vi "Read Data.vi"(7 "SPI Peripheral":refnum<class "SPI Peripheral.lvclass">, 8 "error in (no error)":errorcluster, 9 "Len":u8, 11 "Session In":refnum<class "Session.lvclass">) -> (0 "error out":errorcluster, 1 "Data":string, 3 "Session Out":refnum<class "Session.lvclass">)   [LabVIEW 2020, in "CTI.lvlib" / "SPI Peripheral.lvclass"]
uses:
  SPI Peripheral.lvclass
  Session/Session.lvclass
  SPI Peripheral.lvclass/SPI Peripheral.ctl
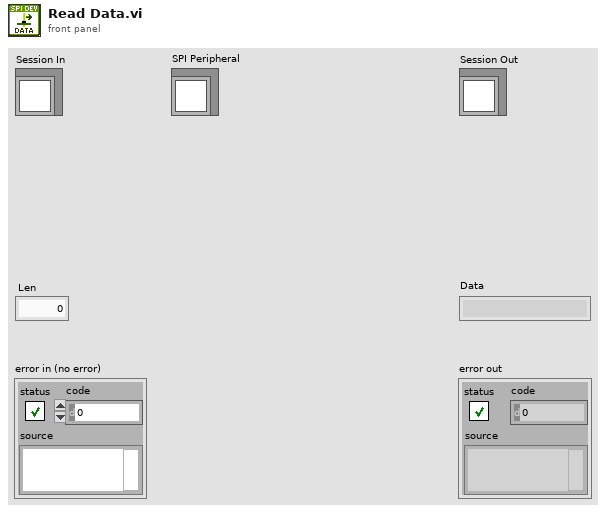
[diagram p1: front panel]
types:
  T1 = typedef "CTI.lvlib/SPI Number.ctl" = i8
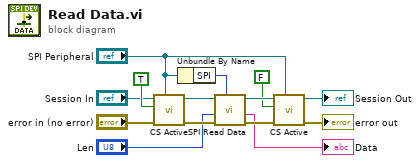
[diagram p0: block diagram]
diagram:
  n1 = call "CS Active.vi"("SPI Peripheral in"="SPI Peripheral", "error in (no error)"="error in (no error)", "CS Active"=TRUE, "Session In"="Session In") -> ("error out"=w12:errorcluster, "Session Out"=w8:refnum<class "Session.lvclass">)  [unwired: 6 in]
  n2 = Unbundle By Name("SPI Peripheral") -> ("SPI"=w11:T1)
  n3 = call "SPI Read Data.vi"("SPI #"=w11, "error in (no error)"=w12, "Len"="Len", "Session in"=w8) -> ("error out"=w13:errorcluster, "Data"=→"Data":string, "Session out"=w14:refnum<class "Session.lvclass">)  [unwired: 5 in]
  n4 = call "CS Active.vi"("SPI Peripheral in"="SPI Peripheral", "error in (no error)"=w13, "CS Active"=FALSE, "Session In"=w14) -> ("error out"=→"error out":errorcluster, "Session Out"=→"Session Out":refnum<class "Session.lvclass">)  [unwired: 6 in]
